vi "read.vi"(8 "error in (no error)":errorcluster, 10 "ILC":refnum<class "ILC.lvclass">, 11 "ReadILCLIMSW1Strategy in":refnum<class "ReadILCDCAAmp2FailStrategy.lvclass">) -> (0 "error out":errorcluster, 2 "Value":dbl, 3 "ReadILCLIMSW1Strategy out":refnum<class "ReadILCDCAAmp2FailStrategy.lvclass">)   [LabVIEW 2015, in "ReadILCDCAAmp2FailStrategy.lvclass"]
uses:
  ReadILCDCAAmp2FailStrategy.lvclass
  <userlib>/Common/ILC/ILC/ILC.lvclass
  <userlib>/Common/ILC/ILC/ILC.lvclass/ILC.ctl
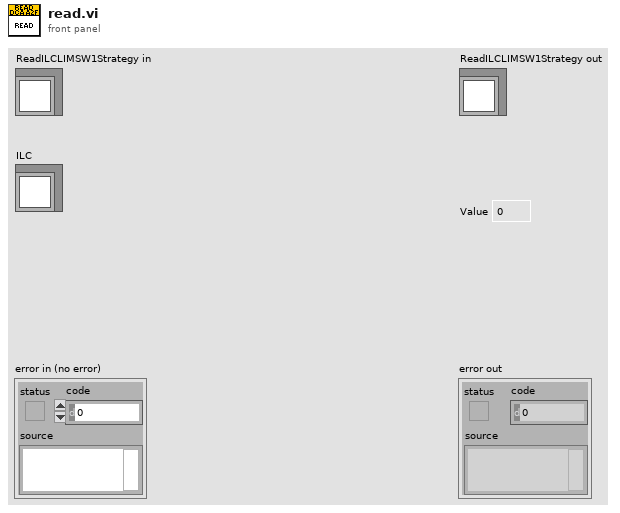
[diagram p1: front panel]
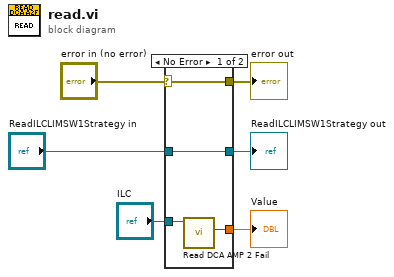
[diagram p0: block diagram]
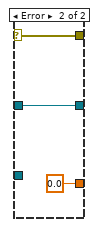
[diagram p2: hidden frame]
diagram:
  n1 = case shown="No Error" "error in (no error)" {
    selector: "error in (no error)" -> [w9 w13]
    tunnel: [w9 w13] -> w5
    tunnel: [w10 w12] -> w3
    tunnel: "ReadILCLIMSW1Strategy in" -> [w10 w12]
    tunnel: [w7 0.0 ("Value")] -> w2
    tunnel: "ILC" -> [w8 _]
    frame No Error {
      n2 = call <userlib>:"Read DCA AMP 2 Fail.vi"("ILC in"=w8) -> ("DCA AMP 2 Fail"=w7:u16)  [unwired: 9 in, 1 out]
    }
    frame Error {
    }
  }
  "error out" <- w5
  "ReadILCLIMSW1Strategy out" <- w3
  "Value" <- w2
